vi "Num2byte.vi"(0 "number":u16) -> (1 "Numeric 2":i8, 2 "Numeric":u32)   [LabVIEW 2009]
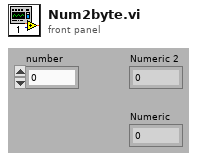
[diagram p1: front panel]
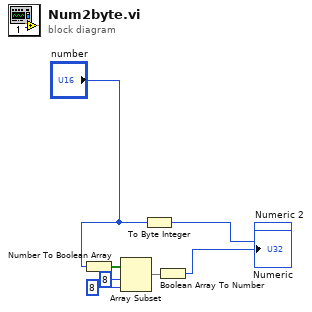
[diagram p0: block diagram]
diagram:
  n1 = Number To Boolean Array(number="number") -> (Boolean array=w2:bool[])
  n2 = Array Subset(array=w2, index=8, length=8) -> (w5:bool[])
  n3 = To Byte Integer(number="number") -> (8bit integer=→"Numeric 2":i8)
  n4 = Boolean Array To Number(Boolean array=w5) -> (number=→"Numeric":u32)
